vi "Move Core.vi"(6 "Relative?":bool, 8 "error in (no error)":errorcluster, 9 "Raw-Position":dbl, 10 "AxisNumber":u8, 11 "CS++IEFWerner in":refnum<class "CS++IEFWerner.lvclass">) -> (0 "error out":errorcluster, 3 "CS++IEFWerner out":refnum<class "CS++IEFWerner.lvclass">)   [LabVIEW 2015, in "CS++IEFWerner.lvlib" / "CS++IEFWerner.lvclass"]
doc: "Starts an absolute or relative movment of an axis."
uses:
  CS++IEFWerner.lvclass
  CS++IEFWerner.lvclass/CS++IEFWerner.ctl
  instr.lib/IEF-pac/IEF Werner.lvlib
  CSPP_DeviceBase/CS++Motor/CS++Motor.lvclass
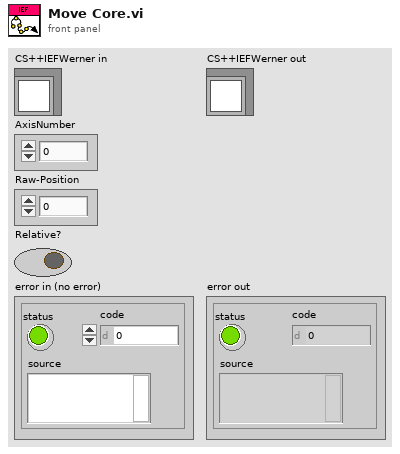
[diagram p1: front panel]
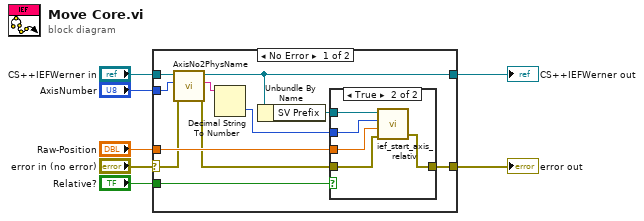
[diagram p0: block diagram]
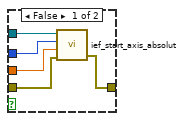
[diagram p2: hidden frame]
diagram:
  n1 = case shown="No Error" "error in (no error)" {
    selector: "error in (no error)" -> [w9 w29]
    tunnel: "CS++IEFWerner in" -> [w13 w30]
    tunnel: "Raw-Position" -> [w17 _]
    tunnel: "AxisNumber" -> [w10 _]
    tunnel: "Relative?" -> [w16 _]
    tunnel: [w15 w29] -> w2
    tunnel: [w12 w30] -> w1
    frame No Error {
      n2 = call "AxisNo2PhysName.vi"("error in (no error)"=w9, "AxisNumber"=w10, "CS++Motor in"=w13) -> ("error out"=w8:errorcluster, "PhysicalChannelName"=w14:string, "CS++Motor out"=w12:refnum<class "CS++IEFWerner.lvclass">)  [unwired: 6 in]
      n3 = Decimal String To Number(string=w14) -> (number=w11:i32)  [unwired: 2 in, 1 out]
      n4 = Unbundle By Name(w12) -> ("SV Prefix"=w18:refnum<k21>)
      n5 = case shown="True" w16 {
        tunnel: w18 -> [w23 w28]
        tunnel: w8 -> [w22 w27]
        tunnel: w17 -> [w21 w26]
        tunnel: w11 -> [w20 w25]
        tunnel: [w19 w24] -> w15
        frame False {
          n6 = call "ief_start_axis_absolut.vi"("error in (no error)"=w22, "Absolute Position"=w21, "Axis Number"=w20, "Tagprefix in"=w23) -> ("error out (no error)"=w19:errorcluster)  [unwired: 2 out]
        }
        frame True {
          n7 = call "ief_start_axis_relativ.vi"("error in (no error)"=w27, "Relative Position"=w26, "Axis Number"=w25, "Tagprefix in"=w28) -> ("error out (no error)"=w24:errorcluster)  [unwired: 2 out]
        }
      }
    }
    frame Error {
    }
  }
  "error out" <- w2
  "CS++IEFWerner out" <- w1
